vi "Logging Message Loop.vi"(7 "Stand alone?":bool=TRUE, 8 "error in (no error)":errorcluster, 9 "Metadata all":T1={"Data Fields"={"operatorName"="LED Life Testing", "project"="LED Life Testing", "measurementType"="", "sphere"="2m (jacketed)", "spectrometer"="", "powerSource"="California Instruments 2253ix", "analyzer"="California Instruments 2253ix", "fixtureType"="NA", "lampType"="A 19", "sourceType"="LED", "testOrientation"="Base Up", "model"="1", "sample"="1", "hours"="1000", "Amp Gain Range"=""}, "Metadata Disable"={"spectrometer"=enum."Disabled and Grayed Out", "sphere"=enum."Disabled and Grayed Out", "analyzer"=enum."Disabled and Grayed Out", "ampGainRange"=enum."Disabled and Grayed Out"}, "Output Path"=path ""}, 10 "Data Queue":refnum<queue>, 11 "Message Queues":T4) -> (0 "error out":errorcluster)   [LabVIEW 2013, in "YKPZ400 Logging.lvlib"]
doc: "The message loop subVI to handle messages pertaining to logging data."
uses:
  YKPZ400 Logging.lvlib
  support/Message Queue/All Message Queues.ctl
  support/Message Queue/Message Cluster.ctl
  electrical2.ctl
  Metadata all typedef.ctl
  Metadata typedef.ctl
  Metadata disable typedef.ctl
  Logging Configuration.ctl
  Logging State.ctl
  support/Message Queue/Enqueue Message (Single).vi
  <vilib>/Utility/error.llb/Error Cluster From Error Code.vi
  <vilib>/ErrorRing/Error Ring.xnode
  support/Message Queue/YKPZ400 Message Queue.lvlib
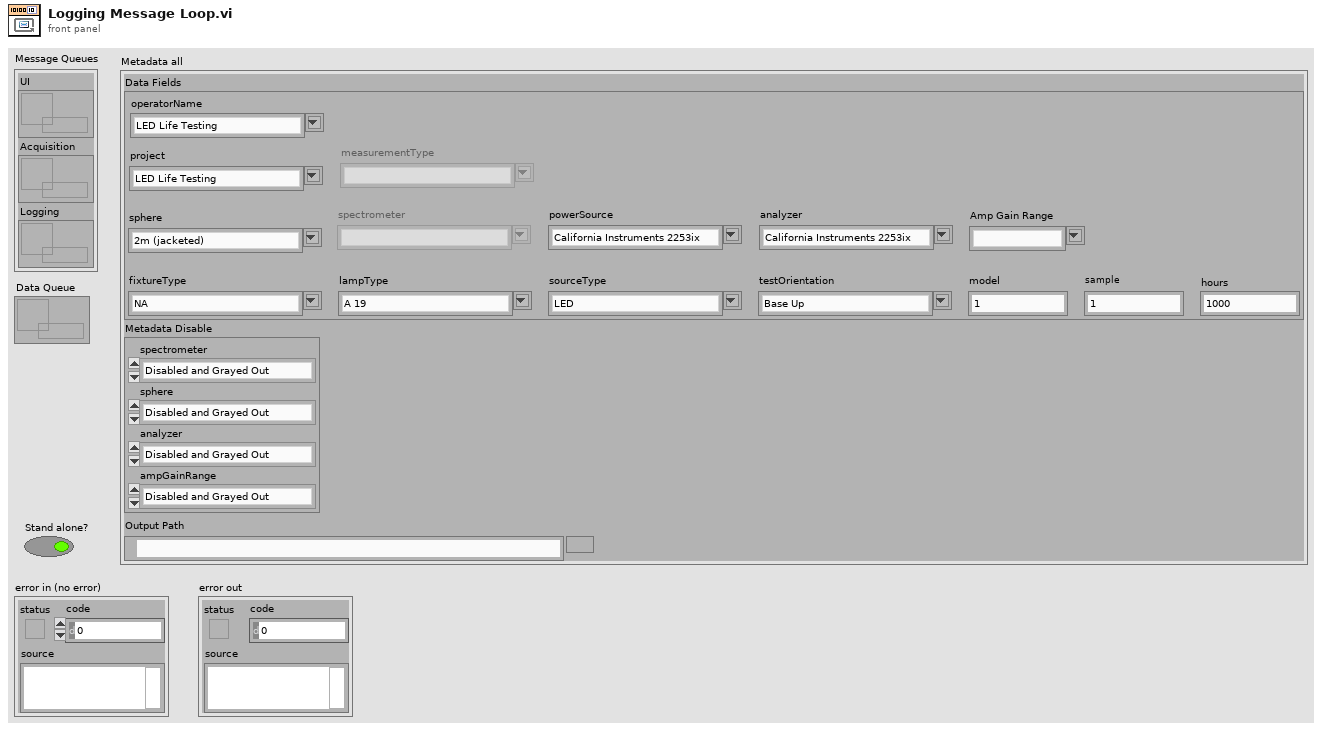
[diagram p1: front panel]
types:
  T1 = typedef "Metadata all typedef.ctl" = cluster{"Data Fields":T2, "Metadata Disable":T3, "Output Path":path}
  T2 = typedef "Metadata typedef.ctl" = cluster{"operatorName":string, "project":string, "measurementType":string, "sphere":string, "spectrometer":string, "powerSource":string, "analyzer":string, "fixtureType":string, "lampType":string, "sourceType":string, "testOrientation":string, "model":string, "sample":string, "hours":string, "Amp Gain Range":string}
  T3 = typedef "Metadata disable typedef.ctl" = cluster{"spectrometer":enum8{"Enabled", "Disabled", "Disabled and Grayed Out"}, "sphere":enum8{"Enabled", "Disabled", "Disabled and Grayed Out"}, "analyzer":enum8{"Enabled", "Disabled", "Disabled and Grayed Out"}, "ampGainRange":enum8{"Enabled", "Disabled", "Disabled and Grayed Out"}}
  T4 = typedef "YKPZ400 Message Queue.lvlib/All Message Queues.ctl" = cluster{"UI":refnum<queue>, "Acquisition":refnum<queue>, "Logging":refnum<queue>}
  T5 = typedef "YKPZ400 Logging.lvlib/Logging Configuration.ctl" = cluster{"Log File Base Path":path, "TDMS File Reference":refnum<k34>, "Module to save":i32}
  T6 = typedef "YKPZ400 Logging.lvlib/Logging State.ctl" = enum16{"Idle", "Logging"}
  T7 = enum16{"open", "open or create", "create or replace", "create", "open (read-only)"}
  T8 = typedef "electrical2.ctl" = cluster{"Time Stamp":timestamp, "Temperature (C)":dbl, "Electrical Data":string[][], "Waveform Graph":waveform(dbl)[]}
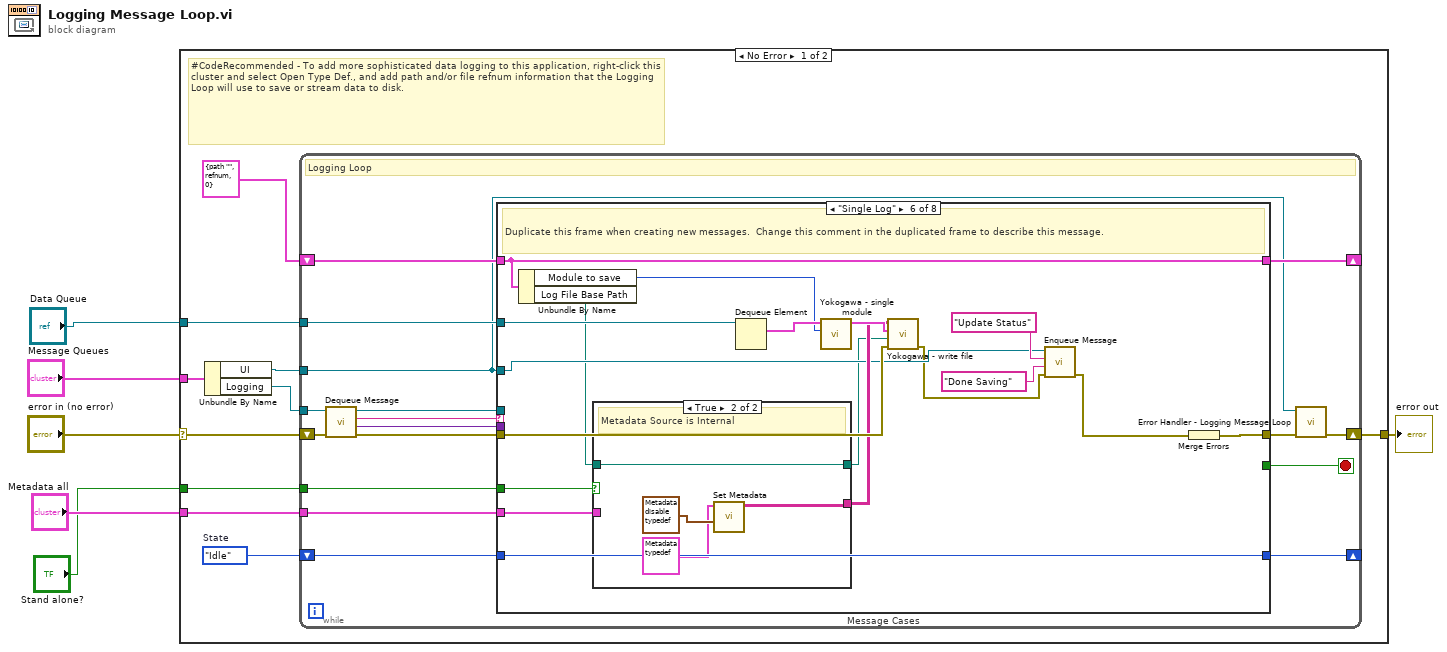
[diagram p0: block diagram]
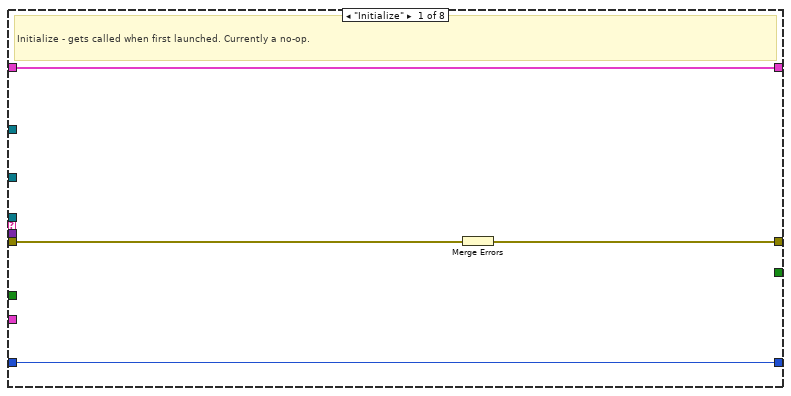
[diagram p2: hidden frame]
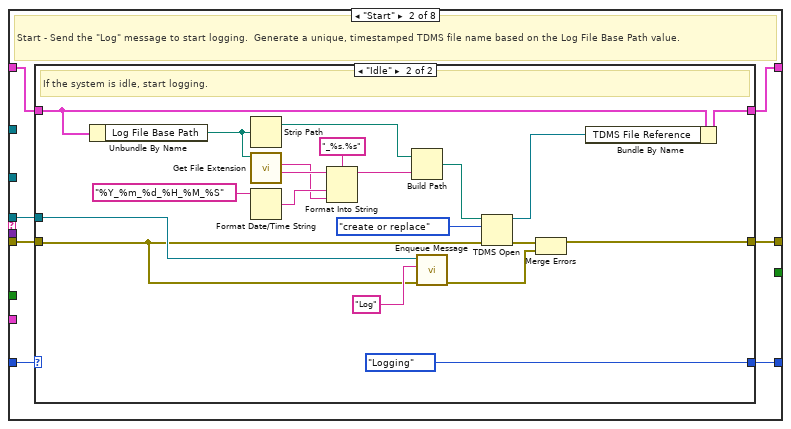
[diagram p3: hidden frame]
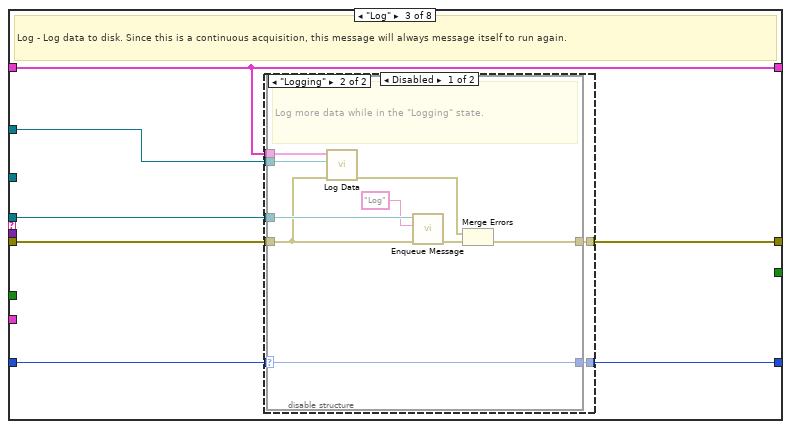
[diagram p5: hidden frame]
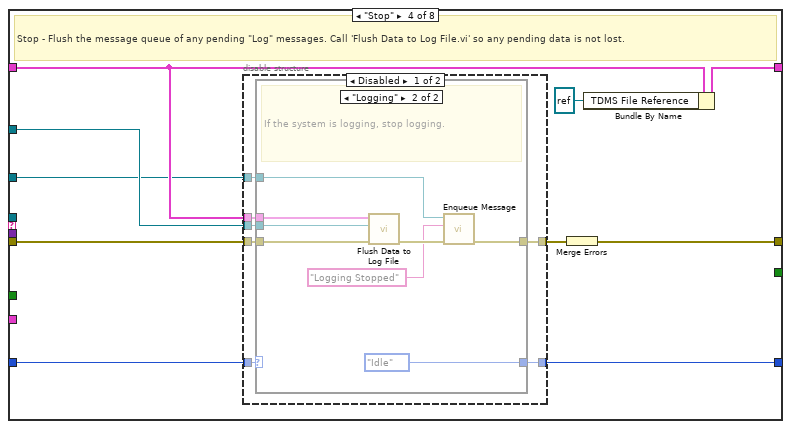
[diagram p8: hidden frame]
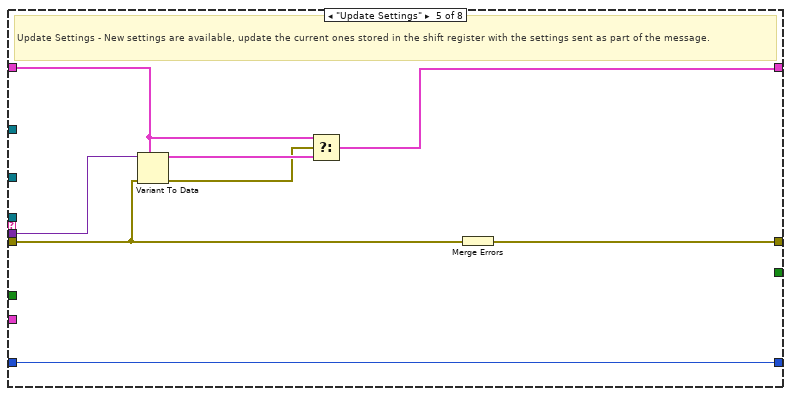
[diagram p11: hidden frame]
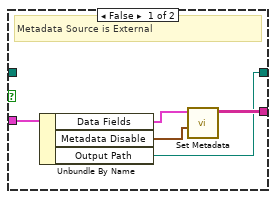
[diagram p12: hidden frame]
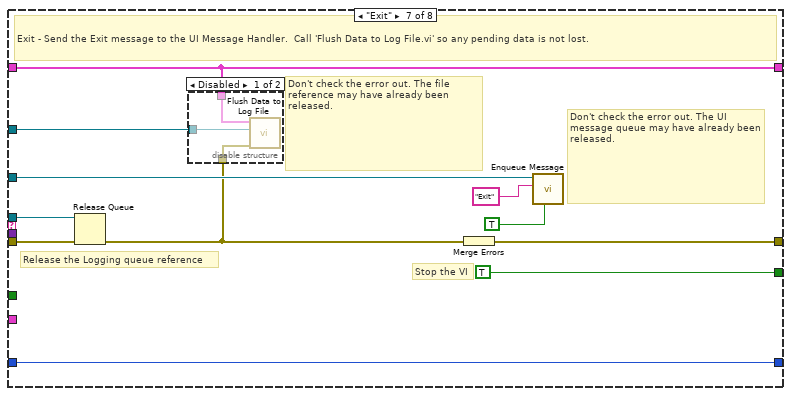
[diagram p13: hidden frame]
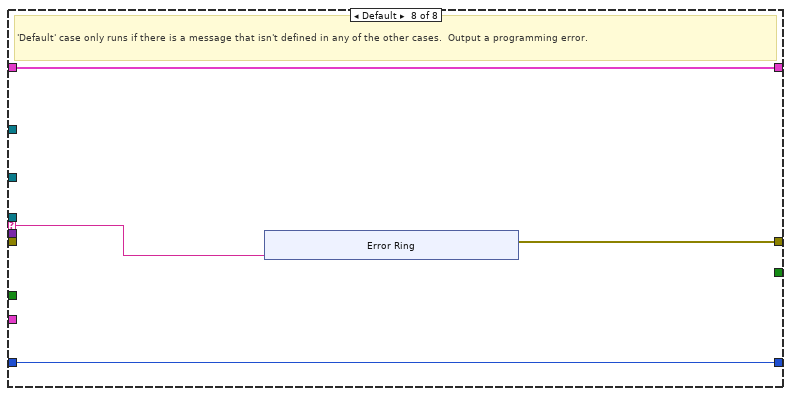
[diagram p15: hidden frame]
diagram:
  n1 = case shown="No Error" "error in (no error)" {
    selector: "error in (no error)" -> [w12 w180]
    tunnel: "Message Queues" -> [w16 _]
    tunnel: [w14 w180] -> w5
    tunnel: "Data Queue" -> [w11 _]
    tunnel: "Metadata all" -> [w8 _]
    tunnel: "Stand alone?" -> [w7 _]
    frame No Error {
      w9 = Logging_State."Idle"  # State
      # "#CodeRecommended - To add more sophisticated data logging to this application, right-click this cluster and select Open Type Def., and add path and/or file refnum information that the Logging Loop will use to save or stream data to disk."
      n2 = Unbundle By Name(w16) -> ("UI"=w10:refnum<queue>, "Logging"=w15:refnum<queue>)
      n3 = while {
        tunnel: w15 -> [w25]
        shift-right: [w32] -> _
        shift-left: T5 {"Log File Base Path"=path "", "TDMS File Reference"=refnum, "Module to save"=0} ("Logging Configuration") -> [w33]
        shift-right: [w21] -> w14
        shift-left: w12 -> [w30]
        tunnel: w10 -> [w19]
        tunnel: w11 -> [w24]
        shift-right: [w22] -> _
        shift-left: w9 -> [w23]
        tunnel: w8 -> [w18]
        tunnel: w7 -> [w17]
        stop <- w31 stop-if-true
        # "Logging Loop"
        n4 = call "Dequeue Message.vi"("error in (no error)"=w30, "Message Queue"=w25) -> ("error out"=w29:errorcluster, "Message Data"=w27:variant, "Message"=w28:string, "dup Message Queue"=w26:refnum<queue>)  [unwired: 6 in]
        n5 = case "Message Cases" shown="\"Single Log\"" w28 {
          selector: w28 -> [_ _ _ _ _ _ _ w169]
          tunnel: w26 -> [_ w43 w73 _ _ _ w159 _]
          tunnel: w29 -> [w35 w42 w71 w96 w121 w138 w162 _]
          tunnel: [w37 w44 w74 w102 w127 w145 w164 w170] -> w20
          tunnel: w33 -> [w36 w41 w70 w97 w125 w140 w157 w172]
          tunnel: [w36 w40 w70 w100 w122 w140 w157 w172] -> w32
          tunnel: [_ _ _ _ _ _ TRUE _] -> w31
          tunnel: w27 -> [_ _ _ _ w126 _ _ _]
          tunnel: w19 -> [_ _ _ w93 _ w135 w163 _]
          tunnel: w24 -> [_ _ w72 w98 _ w143 w156 _]
          tunnel: w23 -> [w34 w39 w69 w95 w120 w144 w155 w171]
          tunnel: [w34 w38 w68 w94 w120 w144 w155 w171] -> w22
          tunnel: w18 -> [_ _ _ _ _ w131 _ _]
          tunnel: w17 -> [_ _ _ _ _ w130 _ _]
          frame "Initialize" {
            # "Initialize - gets called when first launched. Currently a no-op."
            n6 = Merge Errors(w35) -> (w37:errorcluster)
          }
          frame "Start" {
            # "Start - Send the \"Log\" message to start logging.  Generate a unique, timestamped TDMS file name based on the Log File Base Path value."
            n7 = case shown="\"Idle\"" w39 {
              selector: w39 -> [w46 _]
              tunnel: [w45 w49] -> w44
              tunnel: w43 -> [_ w50]
              tunnel: w42 -> [w45 w48]
              tunnel: w41 -> [w47 w51]
              tunnel: [w47 w53] -> w40
              tunnel: [w46 Logging_State."Logging" ("State")] -> w38
              frame "Logging" {
                # "The system is already logging. Ignore the \"Start\" message."
              }
              frame "Idle" {
                # "If the system is idle, start logging."
                n8 = Unbundle By Name(w51) -> ("Log File Base Path"=w66:path)
                n9 = Strip Path(path=w66) -> (stripped path=w63:path)  [unwired: 1 out]
                n10 = call <vilib>:"Get File Extension.vi"("file"=w66) -> ("filename without extension"=w64:string, "lowercase file extension"=w60:string)  [unwired: 7 in, 2 out]
                n11 = Format Date/Time String(time format string (%c)="%Y_%m_%d_%H_%M_%S") -> (date/time string=w61:string)  [unwired: 2 in]
                n12 = Format Into String(format string="_%s.%s", initial string=w64, w61, w60) -> (resulting string=w59:string)  [unwired: 1 in, 1 out]
                n13 = Build Path(base path=w63, name or relative path=w59) -> (appended path=w58:path)
                n14 = call-poly "Enqueue Message.vi"("error in (no error)"=w48, "Message"="Log", "Message Queue"=w50) -> ("error out"=w56:errorcluster)  [unwired: 7 in, 1 out]
                n15 = TDMS Open(8:w48, 10:T7."create or replace" ("operation (0:open)"), 11:w58) -> (0:w57:errorcluster, 3:w54:refnum<k34>)  [unwired: 4 in]
                n16 = Merge Errors(w57, w56) -> (w49:errorcluster)
                n17 = Bundle By Name(cluster=w51, "TDMS File Reference"=w54) -> (w53:T5)
              }
            }
          }
          frame "Log" {
            # "Log - Log data to disk. Since this is a continuous acquisition, this message will always message itself to run again."
            n18 = disable-structure shown="Disabled" {
              disable-tunnel: [w81 _] -> w74
              disable-tunnel: w73 -> [w80 _]
              disable-tunnel: w72 -> [w79 _]
              disable-tunnel: w71 -> [w78 _]
              disable-tunnel: w70 -> [w77 _]
              disable-tunnel: w69 -> [w76 _]
              disable-tunnel: [w75 _] -> w68
              frame Disabled {
                n19 = case shown="\"Logging\"" w76 {
                  selector: w76 -> [w83 w85]
                  tunnel: [w82 w92] -> w81
                  tunnel: w80 -> [_ w90]
                  tunnel: w79 -> [_ w89]
                  tunnel: w78 -> [w82 w84]
                  tunnel: w77 -> [_ w86]
                  tunnel: [w83 w85] -> w75
                  frame "Idle" {
                    # "Ignore \"Log\" messages when the logging is idle."
                  }
                  frame "Logging" {
                    # "Log more data while in the \"Logging\" state."
                    n20 = call "Log Data.vi"("error in (no error)"=w84, "Data Queue"=w89, "Logging Configuration"=w86) -> ("error out"=w88:errorcluster)  [unwired: 8 in]
                    n21 = call-poly "Enqueue Message.vi"("error in (no error)"=w84, "Message"="Log", "Message Queue"=w90) -> ("error out"=w91:errorcluster)  [unwired: 7 in, 1 out]
                    n22 = Merge Errors(w88, w91) -> (w92:errorcluster)
                  }
                }
              }
              frame Enabled {
              }
            }
          }
          frame "Stop" {
            # "Stop - Flush the message queue of any pending \"Log\" messages. Call 'Flush Data to Log File.vi' so any pending data is not lost."
            n23 = disable-structure shown="Disabled" {
              disable-tunnel: [w109 _] -> w101
              disable-tunnel: w98 -> [w108 _]
              disable-tunnel: w97 -> [w107 _]
              disable-tunnel: w96 -> [w106 _]
              disable-tunnel: w95 -> [w105 _]
              disable-tunnel: [w104 _] -> w94
              disable-tunnel: w93 -> [w103 _]
              frame Disabled {
                n24 = case shown="\"Logging\"" w105 {
                  selector: w105 -> [w110 _]
                  tunnel: [w111 w114] -> w109
                  tunnel: w108 -> [_ w118]
                  tunnel: w107 -> [_ w117]
                  tunnel: w106 -> [w111 w116]
                  tunnel: [w110 Logging_State."Idle" ("State")] -> w104
                  tunnel: w103 -> [_ w113]
                  frame "Idle" {
                    # "The system is already idle. Ignore the \"Stop\" message."
                  }
                  frame "Logging" {
                    # "If the system is logging, stop logging."
                    n25 = call "Flush Data to Log File.vi"("error in (no error)"=w116, "Data Queue"=w118, "Logging Configuration"=w117) -> ("error out"=w119:errorcluster)  [unwired: 8 in]
                    n26 = call-poly "Enqueue Message.vi"("error in (no error)"=w119, "Message"="Logging Stopped", "Message Queue"=w113) -> ("error out"=w114:errorcluster)  [unwired: 7 in, 1 out]
                  }
                }
              }
              frame Enabled {
              }
            }
            n27 = Merge Errors(w101) -> (w102:errorcluster)
            n28 = Bundle By Name(cluster=w97, "TDMS File Reference"=refnum<k34> refnum) -> (w100:T5)
          }
          frame "Update Settings" {
            # "Update Settings - New settings are available, update the current ones stored in the shift register with the settings sent as part of the message."
            n29 = Variant To Data(error in=w121, type=w125, Variant=w126) -> (data=w124:T5, error out=w123:errorcluster)
            n30 = Select(t=w125, s=w123, f=w124) -> (s? t:f=w122:T5)
            n31 = Merge Errors(w121) -> (w127:errorcluster)
          }
          frame "Single Log" {
            # "Duplicate this frame when creating new messages.  Change this comment in the duplicated frame to describe this message."
            n32 = Unbundle By Name(w140) -> ("Module to save"=w139:i32, "Log File Base Path"=w129:path)
            n33 = case shown="True" w130 {
              tunnel: [w150 w154] -> w137
              tunnel: w131 -> [w149 _]
              tunnel: w129 -> [_ w151]
              tunnel: [w146 w151] -> w128
              frame False {
                # "Metadata Source is External"
                n34 = Unbundle By Name(w149) -> ("Data Fields"=w148:T2, "Metadata Disable"=w147:T3, "Output Path"=w146:path)
                n35 = call "Set Metadata.vi"("Metadata Disable"=w147, "Data Fields"=w148) -> ("Metadata Out"=w150:string[][])  [unwired: 9 in]
              }
              frame True {
                # "Metadata Source is Internal"
                n36 = call "Set Metadata.vi"("Metadata Disable"=T3 {"spectrometer"=enum."Disabled and Grayed Out", "sphere"=enum."Disabled and Grayed Out", "analyzer"=enum."Enabled", "ampGainRange"=enum."Disabled and Grayed Out"}, "Data Fields"=T2 {"operatorName"="", "project"="", "measurementType"="", "sphere"="", "spectrometer"="", "powerSource"="", "analyzer"="Yokogawa", "fixtureType"="", "lampType"="", "sourceType"="", "testOrientation"="", "model"="", "sample"="", "hours"="", "Amp Gain Range"=""}) -> ("Metadata Out"=w154:string[][])  [unwired: 9 in]
              }
            }
            n37 = Dequeue Element(queue=w143) -> (element=w142:T8)  [unwired: 2 in, 3 out]
            n38 = call "Yokogawa - single module.vi"("Module to save"=w139, "Electrical Data Out in"=w142) -> ("Electrical Data Out out"=w141:T8)  [unwired: 9 in]
            n39 = call "Yokogawa - write file.vi"("error in (no error)"=w138, "Logging Path"=w128, "Electrical Data 2"=w141, "Metadata"=w137) -> ("error out"=w133:errorcluster)  [unwired: 6 in, 1 out]
            n40 = call-poly "Enqueue Message.vi"("error in (no error)"=w133, "Message Data"="Done Saving" ("Message"), "Message"="Update Status", "Message Queue"=w135) -> ("error out"=w132:errorcluster)  [unwired: 6 in, 1 out]
            n41 = Merge Errors(w132) -> (w145:errorcluster)
          }
          frame "Exit" {
            # "Don't check the error out. The file reference may have already been released."
            # "Release the Logging queue reference"
            # "Don't check the error out. The UI message queue may have already been released."
            # "Stop the VI"
            # "Exit - Send the Exit message to the UI Message Handler.  Call 'Flush Data to Log File.vi' so any pending data is not lost."
            n42 = Release Queue(queue=w159, error in (no error)=w162) -> (error out=w158:errorcluster)  [unwired: 1 in, 2 out]
            n43 = disable-structure shown="Disabled" {
              disable-tunnel: w158 -> [w168 _]
              disable-tunnel: w157 -> [w167 _]
              disable-tunnel: w156 -> [w166 _]
              frame Disabled {
                n44 = call "Flush Data to Log File.vi"("error in (no error)"=w168, "Data Queue"=w166, "Logging Configuration"=w167) -> ()  [unwired: 8 in, 1 out]
              }
              frame Enabled {
              }
            }
            n45 = Merge Errors(w158) -> (w164:errorcluster)
            n46 = call-poly "Enqueue Message.vi"("Priority Message? (F)"=TRUE, "Message"="Exit", "Message Queue"=w163) -> ()  [unwired: 7 in, 2 out]
          }
          frame Default {
            # "'Default' case only runs if there is a message that isn't defined in any of the other cases.  Output a programming error."
            n47 = xnode "Error Ring"("parameter 0"=w169) -> ("error out"=w170:errorcluster)
          }
        }
        n48 = call "Error Handler - Logging Message Loop.vi"("error in (no error)"=w20, "Message Queue"=w19) -> ("dup error in"=w21:errorcluster)  [unwired: 8 in, 1 out]
      }
    }
    frame Error {
    }
  }
  "error out" <- w5
